vi "About DoorAccess.vi"() -> ()   [LabVIEW 2011]
panel:
  in  "?":bool
  # "Door Access System v0.1\nDesigner : Ares.Chung\n\nNational Instruments Taiwan Corporation, Taiwan Branch \nAres Chung  | 專案工程師 | cho-wu.chung@ni.com | http://ni.com/taiwan | Mobile: 0988-836099\n | 台北分公司TEL : 02-2377-2222 FAX:02-2377-7676 | 新竹辦事處 TEL 03-657-6222 FAX 03-657-6066"
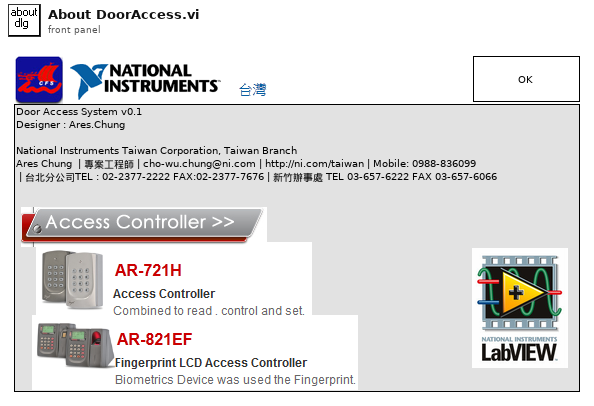
[diagram p1: front panel]
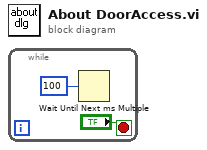
[diagram p0: block diagram]
diagram:
  n1 = while {
    stop <- "?" stop-if-true
    n2 = Wait Until Next ms Multiple(millisecond multiple=u32 100) -> ()  [unwired: 1 out]
  }
